vi "DLPIO20_Close.vi"(11 "VISA resource name":refnum<visa-resource-name>) -> (10 "NoError":bool)   [LabVIEW 2016, in "DLPIO20_PackedLibrary.lvlib"]
uses:
  DLPIO20_PackedLibrary.lvlib
panel:
  out "error out":errorcluster
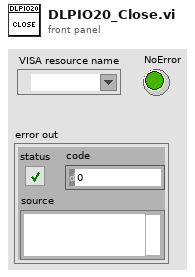
[diagram p1: front panel]
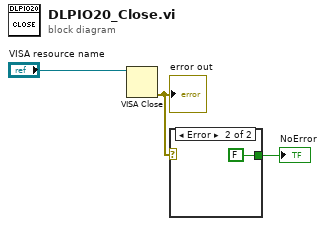
[diagram p0: block diagram]
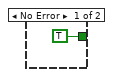
[diagram p2: hidden frame]
diagram:
  n1 = VISA Close(VISA resource name="VISA resource name") -> (error out=w2:errorcluster)  [unwired: 1 in]
  "error out" <- w2
  n2 = case shown="Error" w2 {
    tunnel: [TRUE FALSE] -> w1
    frame No Error {
    }
    frame Error {
    }
  }
  "NoError" <- w1
